vi "NI6071E.ReadData.vi"(0 "i ref in":refnum<vi>, 1 "Use attribute data (f)":bool, 2 "NI6071E Read":T3={"time limit in sec (-1:auto calculate)"=1.0, "number of scans to read (-1:all)"=-1} {"time limit in sec (-1:auto calculate)" format="%0.2f"}, 4 "timeout ms (60000)":i32=60000, 5 "error in (no error)":errorcluster) -> (14 "i ref out":refnum<vi>, 16 "Waveforms":waveform(dbl)[](array[waveform]), 19 "error out":errorcluster)   [LabVIEW 2014, in "NI6071E.lvlib"]
uses:
  NI6071E.lvlib
  NI6071ERead.ctl
  NI6071ECommandCluster.ctl
  NI6071ECommand.ctl
panel:
  in  "Measurement":waveform(dbl)[](graph) caption="Measurement data"
  in  "PPMA Command":T1=enum."ConfigureDAQ"
  in  "PPMA Command Cluster":T2
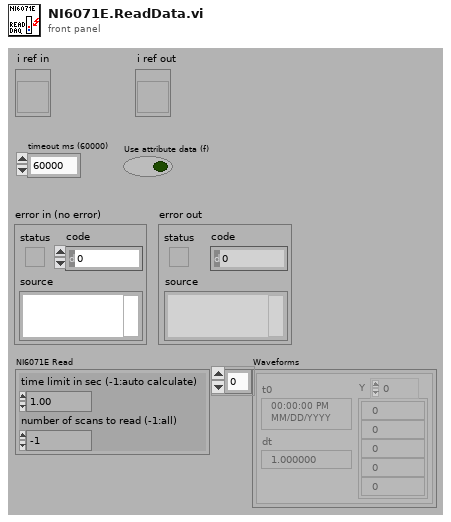
[diagram p1: front panel]
types:
  T1 = typedef "NI6071E.lvlib/NI6071ECommand.ctl" = enum16{"Ping", "Reset", "ConfigureDAQ", "StartDAQ", "StopDAQ", "GetDAQStatus", "ReadData", "SaveData", "CloseConnection"}
  T2 = typedef "NI6071E.lvlib/NI6071ECommandCluster.ctl" = cluster{"Command":string, "Data":string, "error out":errorcluster}
  T3 = typedef "NI6071E.lvlib/NI6071ERead.ctl" = cluster{"time limit in sec (-1:auto calculate)":sgl, "number of scans to read (-1:all)":i32}
  T4 = typedef "NI6071E.lvlib/NI6071E.i attribute.ctl" = cluster{"NI6071E Server":string, "Port":u16, "NI6071E Config":T5, "NI6071E Start":T6, "Waveforms":waveform(dbl)[], "RT Error":errorcluster, "NI6071E Read":T3, "connection ID":refnum<k5>, "DAQ Status":string, "device (1)":i16, "DAQ Status Service ID":i32}
  T5 = typedef "NI6071E.lvlib/NI6071EConfig.ctl" = cluster{"device (1)":i16, "channels (0)":tag[], "buffer size (1000 scans)":i32, "[number of buffers] (1)":i32, "measurement mode structure":cluster{"measurement mode":u16, "reserved":u32}, "input limits (no change)":cluster{"high limit (0.0)":sgl, "low limit (0.0)":sgl}[], "coupling & input config (no change:0)":cluster{"coupling (no change:0)":enum16{"no change", "DC", "AC", "GND", "internal ref."}, "input config (no change:0)":u16}[]}
  T6 = typedef "NI6071E.lvlib/NI6071EStart.ctl" = cluster{"scan rate (40000 scans/sec)":sgl, "trigger type (analog)":enum16{"no trigger", "analog", "digital A", "digital A & B", "scan clock gate"}, "edge or slope \n(rising)":enum16{"no change", "rising", "falling"}, "number of buffers to acquire (1)":i32, "analog chan (PFI0) & level (2.00)":cluster{"trigger channel (empty)":string, "level (0.0)":sgl}, "[additional trig params]":cluster{"hysteresis (0.0)":sgl, "coupling (no change:0)":enum16{"no change", "DC", "AC"}, "delay (0 sec)":sgl, "skip count (0)":i32, "time limit (0 sec)":sgl}}
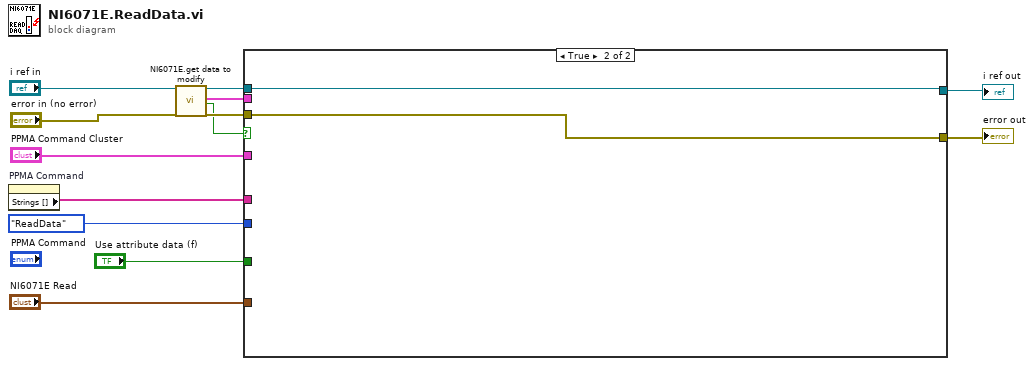
[diagram p0: block diagram]
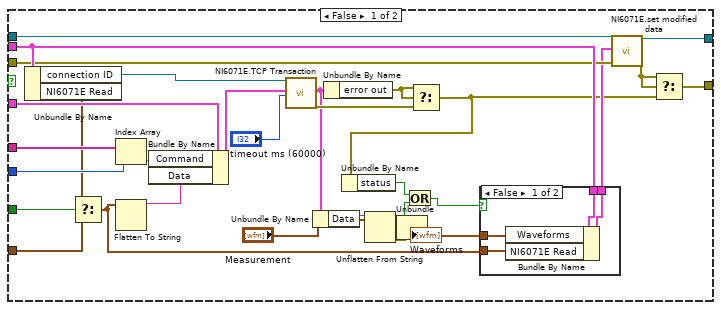
[diagram p2: hidden frame]
diagram:
  n1 = property on="PPMA Command" class="Enum (strict)"() -> ("Strings []"=w5:string[])  [unwired: 2 in, 2 out]
  n2 = call "NI6071E.get data to modify.vi"("i ref in"="i ref in", "error in (no error)"="error in (no error)") -> ("i ref out"=w9:refnum<vi>, "i attribute"=w11:T4, "timed out"=w1:bool, "error out"=w10:errorcluster)  [unwired: 14 in]
  n3 = case shown="True" w1 {
    tunnel: w11 -> [w43 _]
    tunnel: w10 -> [w42 w49]
    tunnel: w9 -> [w41 w50]
    tunnel: [w40 w50] -> w8
    tunnel: [w38 w49] -> w7
    tunnel: "PPMA Command Cluster" -> [w35 _]
    tunnel: w5 -> [w33 _]
    tunnel: NI6071ECommand."ReadData" ("PPMA Command") -> [w32 _]
    tunnel: "Use attribute data (f)" -> [w17 _]
    tunnel: "NI6071E Read" -> [w16 _]
    frame False {
      n4 = Unbundle By Name(w43) -> ("connection ID"=w36:refnum<k5>, "NI6071E Read"=w18:T3)
      n5 = Select(t=w18, s=w17, f=w16) -> (s? t:f=w15:T3)
      n6 = Index Array(array=w33, index=w32) -> (element=w31:string)
      n7 = Flatten To String(anything=w15) -> (data string=w30:string)  [unwired: 3 in, 2 out]
      n8 = Bundle By Name(cluster=w35, "Command"=w31, "Data"=w30) -> (w34:T2)
      n9 = call "NI6071E.TCP Transaction.vi"("connection ID in"=w36, "NI6071E Command Cluster"=w34, "timeout ms (25000)"="timeout ms (60000)") -> ("NI6071E Response"=w26:T2, "error out"=w27:errorcluster)  [unwired: 14 in, 1 out]
      n10 = Unbundle By Name(w26) -> ("Data"=w25:string)
      n11 = Unbundle By Name(w26) -> ("error out"=w28:errorcluster)
      n12 = Unflatten From String(type="Measurement", binary string=w25) -> (value=w20:waveform(dbl)[], error out=w14:errorcluster)  [unwired: 3 in, 1 out]
      "Waveforms" <- w20
      n13 = Unbundle(w14) -> ("status"=w22:bool)  [unwired: 2 out]
      n14 = Select(t=w28, s=w28, f=w27) -> (s? t:f=w24:errorcluster)
      n15 = Unbundle By Name(w24) -> ("status"=w23:bool)
      n16 = Or(x=w23, y=w22) -> (x .or. y?=w21:bool)
      n17 = case shown="False" w21 {
        tunnel: w43 -> [w47 w48]
        tunnel: [w46 w48] -> w37
        tunnel: w15 -> [w45 _]
        tunnel: w20 -> [w44 _]
        frame False {
          n18 = Bundle By Name(cluster=w47, "Waveforms"=w44, "NI6071E Read"=w45) -> (w46:T4)
        }
        frame True {
        }
      }
      n19 = call "NI6071E.set modified data.vi"("i ref in"=w41, "i attribute"=w37, "error in (no error)"=w42) -> ("i ref out"=w40:refnum<vi>, "error out"=w39:errorcluster)  [unwired: 15 in]
      n20 = Select(t=w39, s=w39, f=w24) -> (s? t:f=w38:errorcluster)
    }
    frame True {
    }
  }
  "i ref out" <- w8
  "error out" <- w7
